vi "Amp_Bypass_Switch(S6).vi"(8 "error in":errorcluster, 11 "AMP Function":enum16{"Bypass Amp", "Include Amp"}(ring)) -> (0 "error out":errorcluster, 3 "Verfied":bool)   [LabVIEW 2012]
panel:
  # "Amp Bypass Switch (S6)"
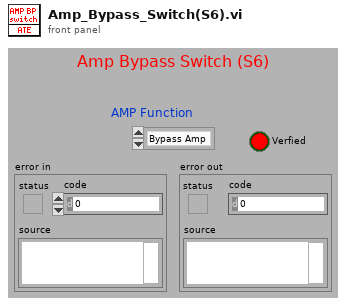
[diagram p1: front panel]
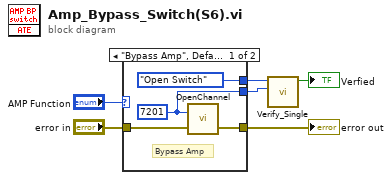
[diagram p0: block diagram]
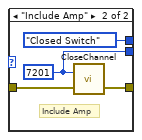
[diagram p2: hidden frame]
diagram:
  n1 = case shown="\"Bypass Amp\", Default" "AMP Function" {
    tunnel: "error in" -> [w10 w14]
    tunnel: [w9 w13] -> w4
    tunnel: [w8 w11] -> w3
    tunnel: [enum16{"Open Switch", "Closed Switch"}."Open Switch" ("Switch Functin") enum16{"Open Switch", "Closed Switch"}."Closed Switch" ("Switch Functin")] -> w2
    frame "Bypass Amp", Default {
      w8 = 7201
      # "Bypass Amp"
      n2 = call "OpenChannel.vi"("error in (no error)"=w10, "Channel ID"=w8) -> ("error out"=w9:errorcluster)  [unwired: 1 in]
    }
    frame "Include Amp" {
      w11 = 7201
      # "Include Amp"
      n3 = call "CloseChannel.vi"("error in (no error)"=w14, "Channel ID"=w11) -> ("error out"=w13:errorcluster)  [unwired: 1 in]
    }
  }
  "error out" <- w4
  n4 = call "Verify_Single.vi"("Switch ID"=w3, "Switch Functin"=w2) -> ("Verfied"=→"Verfied":bool)  [unwired: 8 in, 1 out]
